vi "AH read data.vi"(8 "error in (no error)":errorcluster, 11 "VISA Resource Name":refnum<visa-resource-name>) -> (0 "error out":errorcluster, 1 "Loss":dbl, 2 "Capacitance":dbl, 3 "VISA Resource Name Out":refnum<visa-resource-name>)   [LabVIEW 2016]
panel:
  in  "address":i16
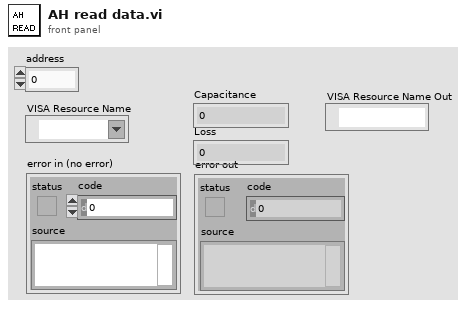
[diagram p1: front panel]
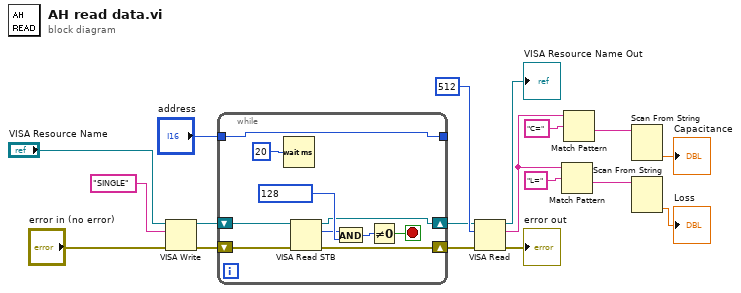
[diagram p0: block diagram]
diagram:
  n1 = VISA Write(VISA resource name="VISA Resource Name", write buffer="SINGLE", error in (no error)="error in (no error)") -> (VISA resource name out=w4:refnum<visa-resource-name>, error out=w12:errorcluster)  [unwired: 1 out]
  n2 = while {
    tunnel: "address" -> [w22]
    shift-right: [w23] -> w8
    shift-left: w12 -> [w28]
    tunnel: [w22] -> _
    shift-right: [w20] -> w3
    shift-left: w4 -> [w21]
    stop <- w25 stop-if-true
    n3 = Wait (ms)(milliseconds to wait=u32 20) -> ()  [unwired: 1 out]
    n4 = VISA Read STB(8:w28, 11:w21) -> (0:w23:errorcluster, 2:w19:u16, 3:w20:refnum<visa-resource-name>)
    n5 = And(x=w19, y=u16 128) -> (x .and. y?=w26:u16)
    n6 = Not Equal To 0?(x=w26) -> (x != 0?=w25:bool)
  }
  n7 = VISA Read(VISA resource name=w3, byte count=u32 512 ("read count"), error in (no error)=w8) -> (VISA resource name out=→"VISA Resource Name Out":refnum<visa-resource-name>, read buffer=w2:string, error out=→"error out":errorcluster)  [unwired: 1 out]
  n8 = Match Pattern(string=w2, regular expression="L=") -> (after substring=w14:string)  [unwired: 4 out]
  n9 = Match Pattern(string=w2, regular expression="C=") -> (after substring=w17:string)  [unwired: 4 out]
  n10 = Scan From String(input string=w17) -> (output 1=→"Capacitance":dbl)  [unwired: 3 in, 4 out]
  n11 = Scan From String(input string=w14) -> (output 1=→"Loss":dbl)  [unwired: 3 in, 4 out]
